vi "PFI-28000-Utils_Throw Error.vi"(0 "Error Message":string, 1 "Throw?":bool=TRUE, 5 "Error Code":i32, 11 "error in (no error)":errorcluster) -> (15 "error out":errorcluster)   [LabVIEW 2017, in "PFI-28000-Utils.lvlib"]
uses:
  PFI-28000-Utils.lvlib
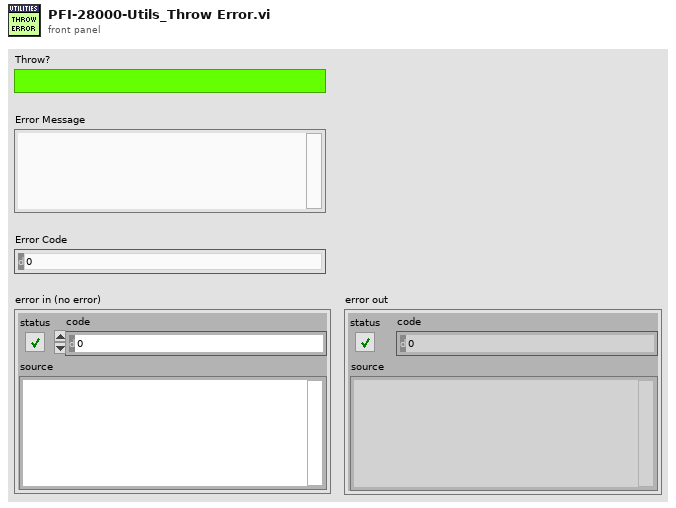
[diagram p1: front panel]
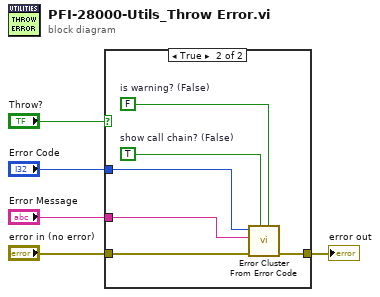
[diagram p0: block diagram]
diagram:
  n1 = case shown="True" "Throw?" {
    tunnel: "Error Message" -> [_ w9]
    tunnel: "error in (no error)" -> [w6 w12]
    tunnel: "Error Code" -> [_ w10]
    tunnel: [w6 w11] -> w2
    frame False {
    }
    frame True {
      w7 = FALSE  # is warning? (False)
      w8 = TRUE  # show call chain? (False)
      n2 = call <vilib>:"Error Cluster From Error Code.vi"("is warning? (False)"=w7, "show call chain? (False)"=w8, "error in (no error)"=w12, "error message (\"\")"=w9, "error code (0)"=w10) -> ("error out"=w11:errorcluster)  [unwired: 4 in]
    }
  }
  "error out" <- w2
